vi "Adjust Sample Size.vi"(11 "Sample Size In":i32) -> (3 "Sample Size Out":i32)   [LabVIEW 2019, in "Audio Processing.lvlib"]
doc: "Ensures the Sample Size is never in the range -1 to 1. Attempting to interpolate an array of 0 or 1 samples generates an audio buffer filled with NaN values."
uses:
  Audio Processing.lvlib
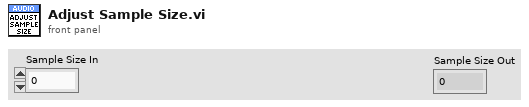
[diagram p1: front panel]
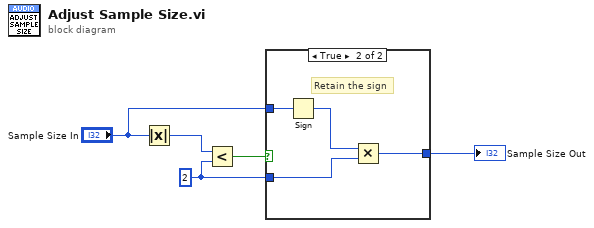
[diagram p0: block diagram]
diagram:
  w4 = 2 ("y")
  n1 = Absolute Value(x="Sample Size In") -> (abs(x)=w2:i32)
  n2 = Less?(x=w2, y=w4) -> (x < y?=w5:bool)
  n3 = case shown="True" w5 {
    tunnel: w4 -> [_ w10]
    tunnel: [w6 w9] -> w3
    tunnel: "Sample Size In" -> [w6 w8]
    frame False {
    }
    frame True {
      # "Retain the sign"
      n4 = Sign(1:w8) -> (0:w7:i32)
      n5 = Multiply(x=w7, y=w10) -> (x*y=w9:i32)
    }
  }
  "Sample Size Out" <- w3
